vi "Concatenate result strings.vi"(7 "Location":enum16{"Start", "End"}(ring), 8 "Message":string, 9 "Description":string, 10 "Status":T1, 11 "Input String":string) -> (3 "Output String":string)   [LabVIEW 2020, in "Method Result.lvlib"]
uses:
  Method Result.lvlib
  Assertion Result/Public/TypeDefs/Status.ctl
  Assertion Result/Assertion Result.lvlib
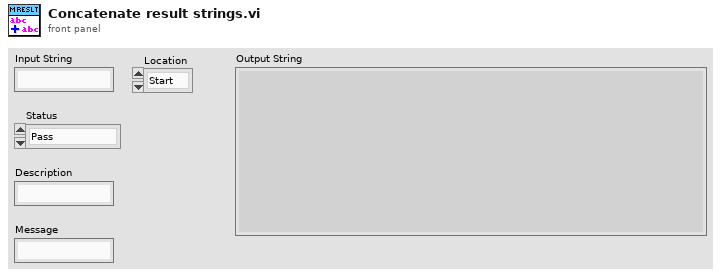
[diagram p1: front panel]
types:
  T1 = typedef "Assertion Result.lvlib/Status.ctl" = enum16{"Pass", "Fail", "Error", "Skipped", "Setup Error", "Broken", "Teardown Error"}
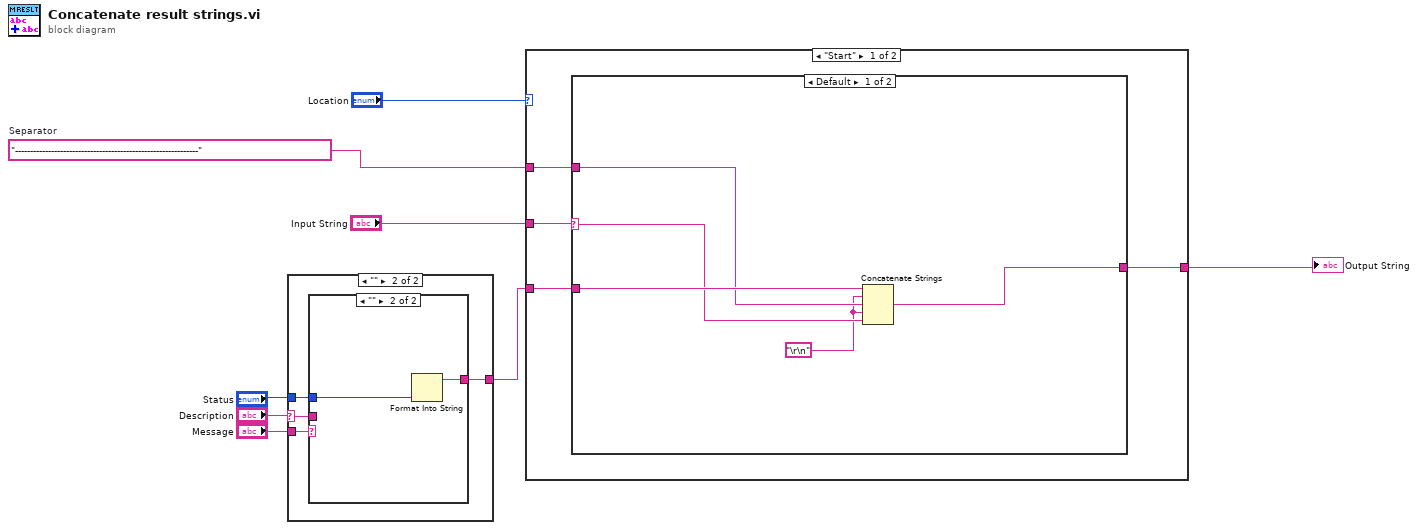
[diagram p0: block diagram]
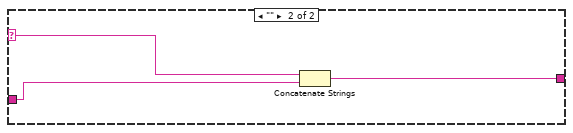
[diagram p2: hidden frame]
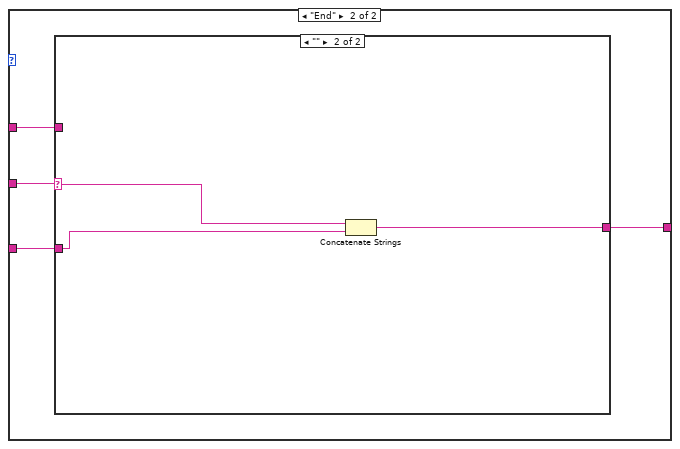
[diagram p3: hidden frame]
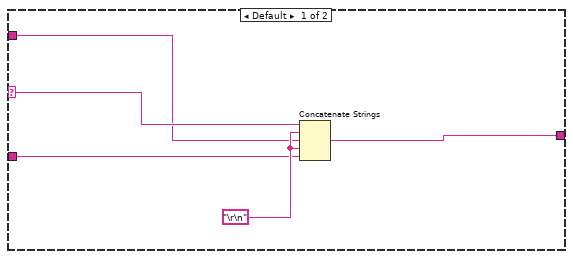
[diagram p4: hidden frame]
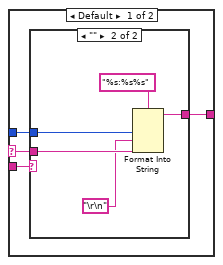
[diagram p5: hidden frame]
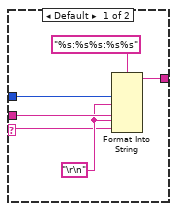
[diagram p6: hidden frame]
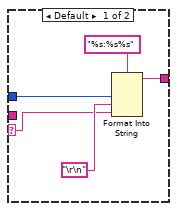
[diagram p7: hidden frame]
diagram:
  w7 = "-------------------------------------------------------------"  # Separator
  n1 = case shown="\"\"" "Description" {
    selector: "Description" -> [w11 w26]
    tunnel: "Status" -> [w12 w27]
    tunnel: "Message" -> [w10 w25]
    tunnel: [w9 w24] -> w2
    frame Default {
      n2 = case shown="\"\"" w10 {
        selector: w10 -> [w15 _]
        tunnel: w12 -> [w18 w22]
        tunnel: w11 -> [w17 w21]
        tunnel: [w14 w19] -> w9
        frame Default {
          w16 = "\r\n"
          n3 = Format Into String(format string="%s:%s%s:%s%s", w18, w16, w17, w16, w15) -> (resulting string=w14:string)  [unwired: 2 in, 1 out]
        }
        frame "" {
          n4 = Format Into String(format string="%s:%s%s", w22, "\r\n", w21) -> (resulting string=w19:string)  [unwired: 2 in, 1 out]
        }
      }
    }
    frame "" {
      n5 = case shown="\"\"" w25 {
        selector: w25 -> [w30 _]
        tunnel: w27 -> [w32 w34]
        tunnel: w26 -> [_ _]
        tunnel: [w29 w33] -> w24
        frame Default {
          n6 = Format Into String(format string="%s:%s%s", w32, "\r\n", w30) -> (resulting string=w29:string)  [unwired: 2 in, 1 out]
        }
        frame "" {
          n7 = Format Into String(w34) -> (resulting string=w33:string)  [unwired: 3 in, 1 out]
        }
      }
    }
  }
  n8 = case shown="\"Start\"" "Location" {
    tunnel: w7 -> [w36 w48]
    tunnel: "Input String" -> [w38 w50]
    tunnel: w2 -> [w37 w49]
    tunnel: [w35 w47] -> w1
    frame "Start" {
      n9 = case shown="Default" w38 {
        selector: w38 -> [w40 w44]
        tunnel: w37 -> [w43 w46]
        tunnel: w36 -> [w42 _]
        tunnel: [w41 w45] -> w35
        frame Default {
          w39 = "\r\n"
          n10 = Concatenate Strings(w43, w39, w42, w39, w40) -> (w41:string)
        }
        frame "" {
          n11 = Concatenate Strings(w44, w46) -> (w45:string)
        }
      }
    }
    frame "End" {
      n12 = case shown="\"\"" w50 {
        selector: w50 -> [w54 w56]
        tunnel: w49 -> [w52 w58]
        tunnel: w48 -> [w51 _]
        tunnel: [w55 w57] -> w47
        frame Default {
          w53 = "\r\n"
          n13 = Concatenate Strings(w54, w53, w51, w53, w52) -> (w55:string)
        }
        frame "" {
          n14 = Concatenate Strings(w56, w58) -> (w57:string)
        }
      }
    }
  }
  "Output String" <- w1
